vi "Getting_TRACE DATA.vi"(6 "Start+timeout?":bool, 8 "error in (no error)":errorcluster, 11 "Class TCP in":T1) -> (0 "error out":errorcluster, 3 "Class TCP out":T1)   [LabVIEW 2022 SP3]
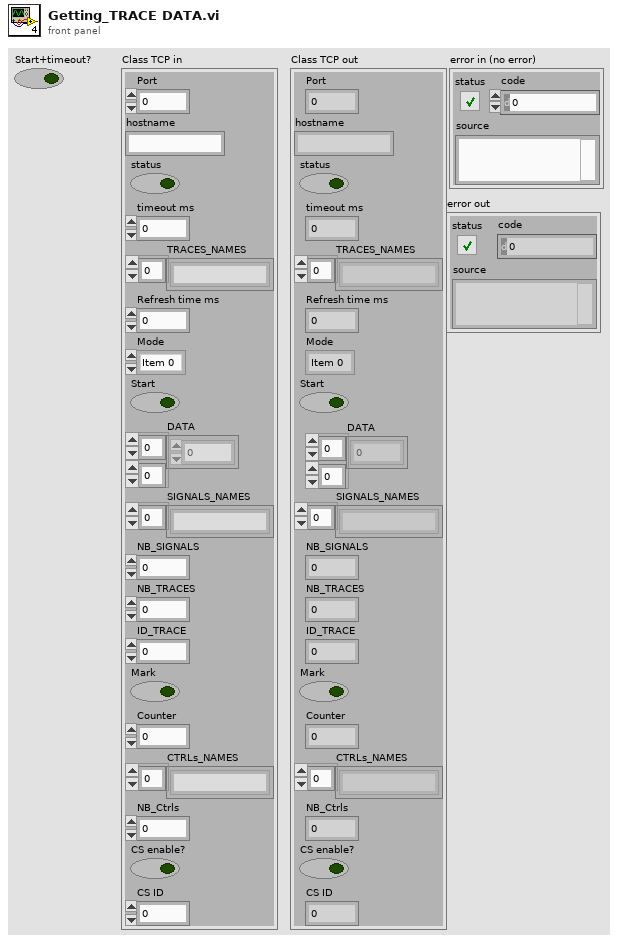
[diagram p1: front panel]
types:
  T1 = cluster{"Port":i32, "hostname":string, "status":bool, "timeout ms":i32, "TRACES_NAMES":string[], "Refresh time ms":i32, "Mode":enum32{"Item 0", "Item 1"}, "Start":bool, "DATA":sgl[][], "SIGNALS_NAMES":string[], "NB_SIGNALS":i32, "NB_TRACES":i32, "ID_TRACE":i32, "Mark":bool, "Counter":i32, "CTRLs_NAMES":string[], "NB_Ctrls":i32, "CS enable?":bool, "CS ID":i32}
  T2 = cluster{"TRACE_SIZE":i32, "CS_ID":i32, "TRACE ID":i32, "CMD":i32, "DATA(M)":i32}
  T3 = cluster{"timeout ms":i32, "remote port":u16, "Address":string}
  T4 = cluster{"SIZE":i32, " TRACE DATA":sgl[], "TRACE_SIZE":i32, "NB_TRACES":i32, "NB_TRACED_SIGNALS":i32, "NAMES TRACED SIGNALS":string[], "NAMES TRACES":string[], "CS STATUS":i32, "NB_CSs":i32, "NAMES CSs":string[], "DATA (M)":sgl[], "CMD":i32}
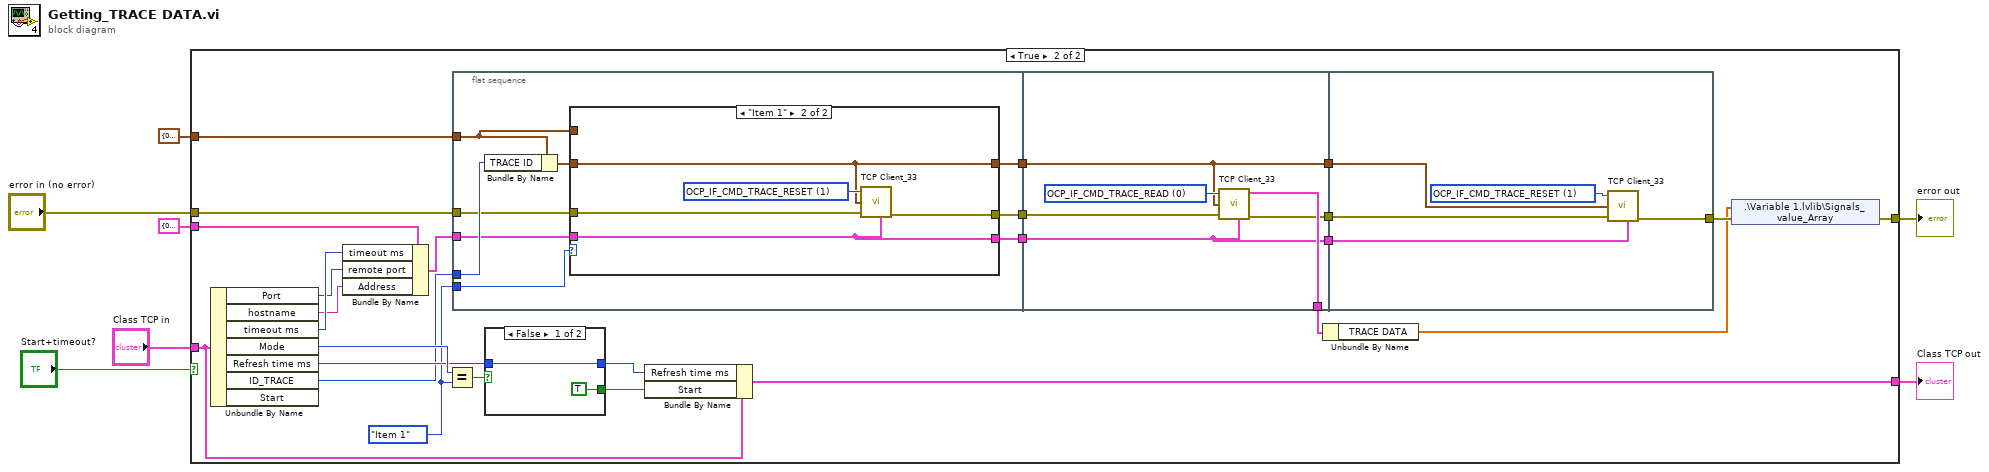
[diagram p0: block diagram]
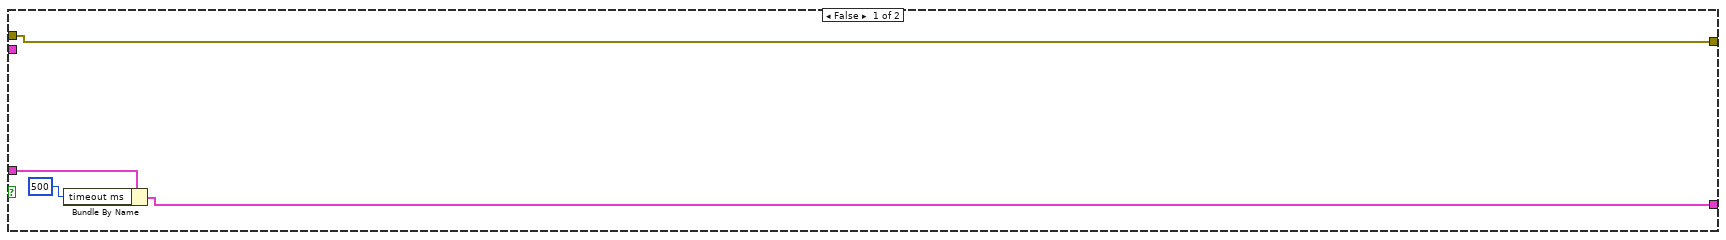
[diagram p2: hidden frame]
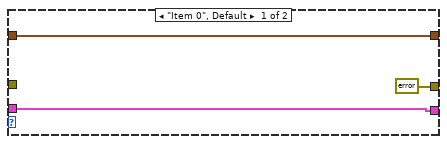
[diagram p3: hidden frame]
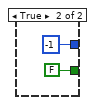
[diagram p4: hidden frame]
diagram:
  n1 = case shown="True" "Start+timeout?" {
    tunnel: "Class TCP in" -> [w11 w18]
    tunnel: [w10 w30] -> w5
    tunnel: T2 {"TRACE_SIZE"=0, "CS_ID"=0, "TRACE ID"=0, "CMD"=0, "DATA(M)"=0} ("Input Cluster") -> [_ w21]
    tunnel: T3 {"timeout ms"=0, "remote port"=0, "Address"=""} ("Comunication Cluster") -> [_ w20]
    tunnel: "error in (no error)" -> [w8 w13]
    tunnel: [w8 w12] -> w1
    frame False {
      n2 = Bundle By Name(cluster=w11, "timeout ms"=500) -> (w10:T1)
    }
    frame True {
      w14 = enum32{"Item 0", "Item 1"}."Item 1" ("Mode")
      n3 = Unbundle By Name(w18) -> ("Port"=w25:i32, "hostname"=w24:string, "timeout ms"=w26:i32, "Mode"=w37:enum32{"Item 0", "Item 1"}, "Refresh time ms"=w35:i32, "ID_TRACE"=w33:i32)  [unwired: 1 out]
      n4 = Bundle By Name(cluster=w20, "timeout ms"=w26, "remote port"=w25, "Address"=w24) -> (w23:T3)
      n5 = Equal?(x=w37, y=w14) -> (x = y?=w36:bool)
      n6 = flat-sequence {
        tunnel: w23 -> [w44]
        tunnel: w21 -> [w40]
        tunnel: w33 -> [w46]
        tunnel: [w45] -> w17
        tunnel: [w43] -> w16
        tunnel: [w42] -> w15
        tunnel: w14 -> [w41]
        tunnel: w13 -> [w38]
        tunnel: [w60] -> w32
        tunnel: [w59] -> w31
        tunnel: [w55] -> w28
        tunnel: [w57] -> w27
        tunnel: w17 -> [w55]
        tunnel: w16 -> [w57]
        tunnel: w15 -> [w56]
        tunnel: w31 -> [w65]
        tunnel: w28 -> [w64]
        tunnel: w27 -> [w63]
        tunnel: [w61] -> w22
        frame #0 {
          n7 = Bundle By Name(cluster=w40, "TRACE ID"=w46) -> (w39:T2)
          n8 = case shown="\"Item 1\"" w41 {
            tunnel: w40 -> [_ _]
            tunnel: [w47 w51] -> w45
            tunnel: w44 -> [w48 w54]
            tunnel: [w48 w54] -> w43
            tunnel: [errorcluster {"status"=FALSE, "code"=0, "source"=""} ("error out") w53] -> w42
            tunnel: w39 -> [w47 w51]
            tunnel: w38 -> [_ w50]
            frame "Item 0", Default {
            }
            frame "Item 1" {
              w52 = 1 items=["OCP_IF_CMD_TRACE_READ", "OCP_IF_CMD_TRACE_RESET", "OCP_IF_CMD_TRACE_GET_SIZE", "OCP_IF_CMD_TRACE_SET_SIZE", "OCP_IF_CMD_TRACE_GET_NUMBER_SIGNALS", "OCP_IF_CMD_TRACE_GET_SIGNALS_NAMES", "OCP_IF_CMD_TRACE_GET_NUMBER_TRACES", "OCP_IF_CMD_TRACE_GET_TRACES_NAMES", "OCP_IF_CMD_TRACE_GET_ADDRESS", "OCP_IF_CMD_CS_STATUS", "OCP_IF_CMD_CS_ENABLE", "OCP_IF_CMD_CS_DISABLE", "OCP_IF_CMD_CS_CONTROLLER_IF", "OCP_IF_CMD_CS_HARDWARE_IF", "OCP_IF_CMD_CS_GET_NUMBER_CONTROLLERS", "OCP_IF_CMD_CS_GET_CONTROLLERS_NAMES", "OCP_IF_CMD_PLATFORM_ID", "OCP_IF_CMD_PLATFORM_IF", "OCP_IF_CMD_OPIL_UPDATE_MEASUREMENTS", "OCP_IF_CMD_OPIL_UPDATE_SIM_DATA", "OCP_IF_CMD_OPIL_RUN_CONTROL", "OCP_IF_CMD_OPIL_INITIALIZE_CONTROL", "OCP_IF_CMD_OPIL_GET_CONTROL", "OCP_IF_CMD_OPIL_GET_CONTROLLER_DATA", "OCP_IF_CMD_END"] ("CMD")
              n9 = call "TCP Client_33.vi"("CMD"=w52, "Input Cluster"=w51, "error in (no error)"=w50, "Comunication Cluster"=w54) -> ("error out"=w53:errorcluster)  [unwired: 4 in, 2 out]
            }
          }
        }
        frame #1 {
          w58 = 0 items=["OCP_IF_CMD_TRACE_READ", "OCP_IF_CMD_TRACE_RESET", "OCP_IF_CMD_TRACE_GET_SIZE", "OCP_IF_CMD_TRACE_SET_SIZE", "OCP_IF_CMD_TRACE_GET_NUMBER_SIGNALS", "OCP_IF_CMD_TRACE_GET_SIGNALS_NAMES", "OCP_IF_CMD_TRACE_GET_NUMBER_TRACES", "OCP_IF_CMD_TRACE_GET_TRACES_NAMES", "OCP_IF_CMD_TRACE_GET_ADDRESS", "OCP_IF_CMD_CS_STATUS", "OCP_IF_CMD_CS_ENABLE", "OCP_IF_CMD_CS_DISABLE", "OCP_IF_CMD_CS_CONTROLLER_IF", "OCP_IF_CMD_CS_HARDWARE_IF", "OCP_IF_CMD_CS_GET_NUMBER_CONTROLLERS", "OCP_IF_CMD_CS_GET_CONTROLLERS_NAMES", "OCP_IF_CMD_PLATFORM_ID", "OCP_IF_CMD_PLATFORM_IF", "OCP_IF_CMD_OPIL_UPDATE_MEASUREMENTS", "OCP_IF_CMD_OPIL_UPDATE_SIM_DATA", "OCP_IF_CMD_OPIL_RUN_CONTROL", "OCP_IF_CMD_OPIL_INITIALIZE_CONTROL", "OCP_IF_CMD_OPIL_GET_CONTROL", "OCP_IF_CMD_OPIL_GET_CONTROLLER_DATA", "OCP_IF_CMD_END"] ("CMD")
          n10 = call "TCP Client_33.vi"("CMD"=w58, "Input Cluster"=w55, "error in (no error)"=w56, "Comunication Cluster"=w57) -> ("Output cluster"=w60:T4, "error out"=w59:errorcluster)  [unwired: 4 in, 1 out]
        }
        frame #2 {
          w62 = 1 items=["OCP_IF_CMD_TRACE_READ", "OCP_IF_CMD_TRACE_RESET", "OCP_IF_CMD_TRACE_GET_SIZE", "OCP_IF_CMD_TRACE_SET_SIZE", "OCP_IF_CMD_TRACE_GET_NUMBER_SIGNALS", "OCP_IF_CMD_TRACE_GET_SIGNALS_NAMES", "OCP_IF_CMD_TRACE_GET_NUMBER_TRACES", "OCP_IF_CMD_TRACE_GET_TRACES_NAMES", "OCP_IF_CMD_TRACE_GET_ADDRESS", "OCP_IF_CMD_CS_STATUS", "OCP_IF_CMD_CS_ENABLE", "OCP_IF_CMD_CS_DISABLE", "OCP_IF_CMD_CS_CONTROLLER_IF", "OCP_IF_CMD_CS_HARDWARE_IF", "OCP_IF_CMD_CS_GET_NUMBER_CONTROLLERS", "OCP_IF_CMD_CS_GET_CONTROLLERS_NAMES", "OCP_IF_CMD_PLATFORM_ID", "OCP_IF_CMD_PLATFORM_IF", "OCP_IF_CMD_OPIL_UPDATE_MEASUREMENTS", "OCP_IF_CMD_OPIL_UPDATE_SIM_DATA", "OCP_IF_CMD_OPIL_RUN_CONTROL", "OCP_IF_CMD_OPIL_INITIALIZE_CONTROL", "OCP_IF_CMD_OPIL_GET_CONTROL", "OCP_IF_CMD_OPIL_GET_CONTROLLER_DATA", "OCP_IF_CMD_END"] ("CMD")
          n11 = call "TCP Client_33.vi"("CMD"=w62, "Input Cluster"=w64, "error in (no error)"=w65, "Comunication Cluster"=w63) -> ("error out"=w61:errorcluster)  [unwired: 4 in, 2 out]
        }
      }
      n12 = case shown="False" w36 {
        tunnel: [TRUE FALSE] -> w34
        tunnel: [w66 i8 -1 ("t")] -> w29
        tunnel: w35 -> [w66 _]
        frame False {
        }
        frame True {
        }
      }
      n13 = Bundle By Name(cluster=w18, "Refresh time ms"=w29, "Start"=w34) -> (w30:T1)
      n14 = Unbundle By Name(w32) -> ("TRACE DATA"=w19:sgl[])
      n15 = shared-variable ".\\Variable 1.lvlib\\Signals_value_Array"(w19, error in=w22) -> (error out=w12:errorcluster)
    }
  }
  "Class TCP out" <- w5
  "error out" <- w1
